vi "Plotter Keyvan.vi"() -> ()   [LabVIEW 2014]
panel:
  out "5":cluster{"Time":dbl[], "yi":dbl[]}[](graph)
  in  "Tab Control":enum32{"Graph 1", "Graph 2"}(tab)
  in  "RR":bool
  in  "RL":bool
  in  "FR":bool
  in  "FL":bool
  in  "RR":bool
  in  "RL":bool
  in  "FR":bool
  in  "FL":bool
  out "4":cluster{"Time":dbl[], "yi":dbl[]}[](graph)
  out "3":cluster{"Time":dbl[], "Vbb2":dbl[]}(graph)
  out "2":cluster{"Time":dbl[], "Vbb2":dbl[]}(graph)
  out "1":cluster{"Time":dbl[], "Vbb2":dbl[]}(graph)
  in  "Play Button":bool
  in  "Process Stop Button":bool
  in  "File path":path
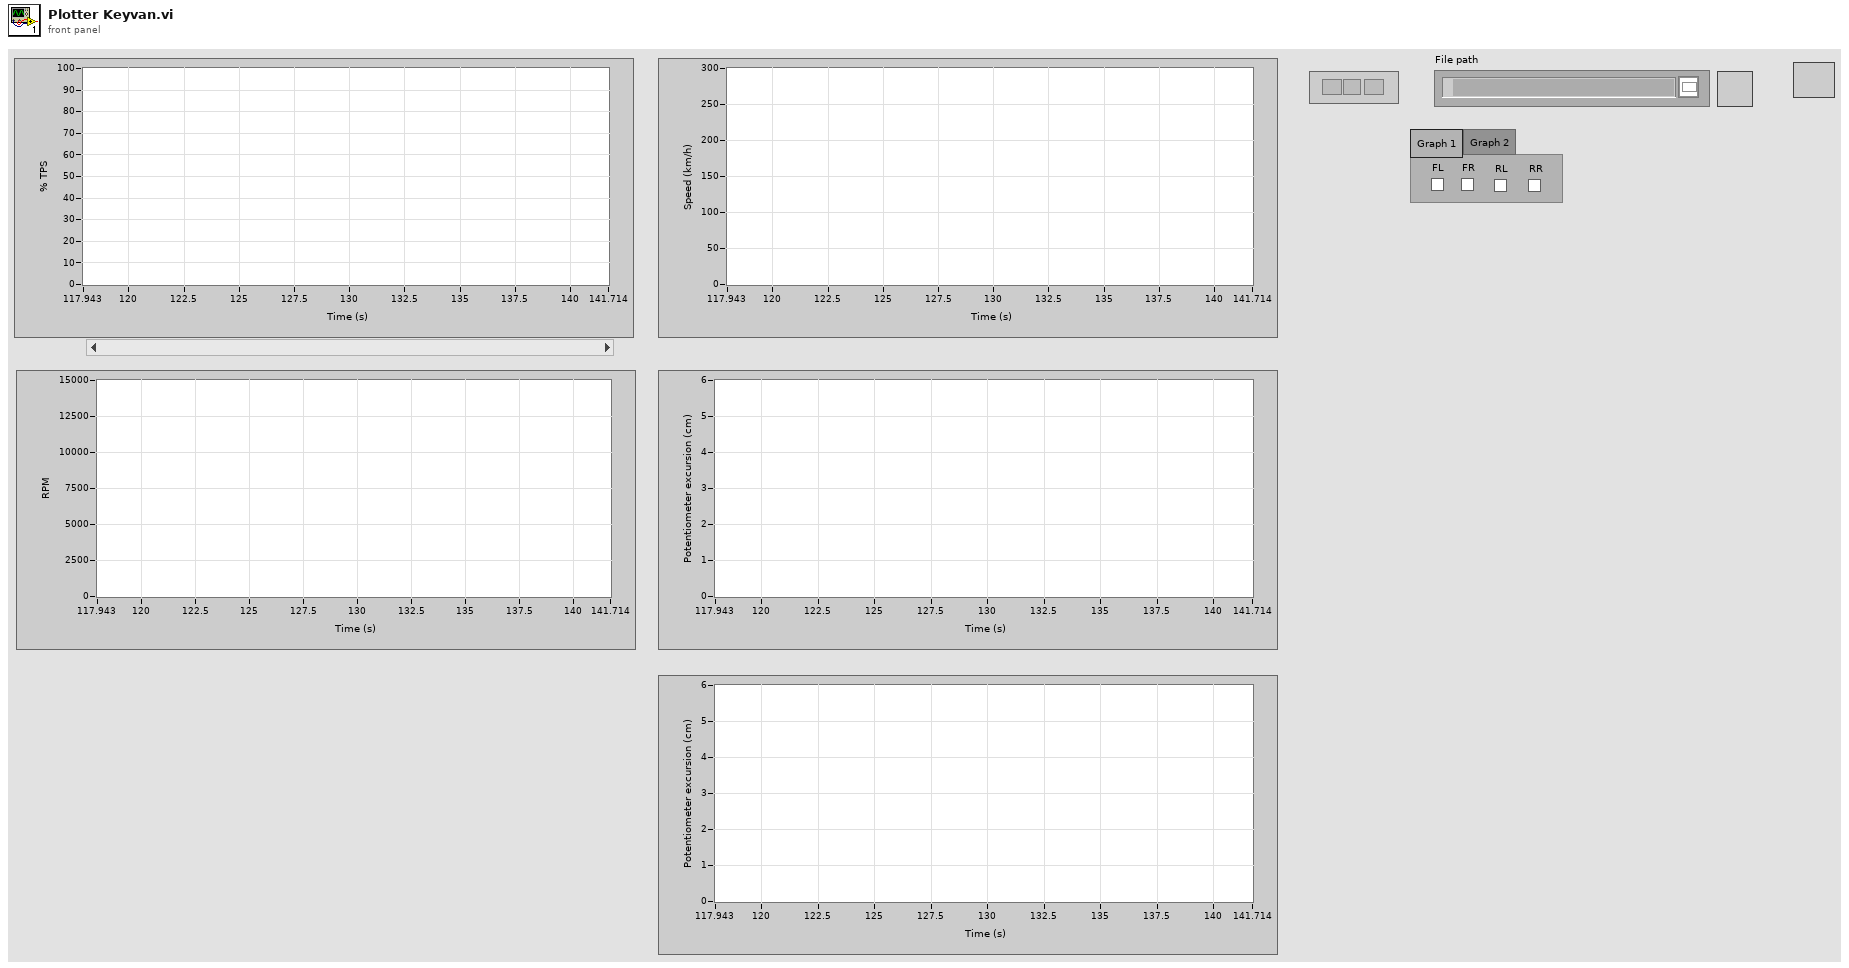
[diagram p1: front panel]
types:
  T1 = typedef "CAR Data Cluster.ctl" = cluster{"revs":dbl[], "rev/min":dbl[], "TPS":dbl[], "map":dbl[], "T H20":dbl[], "T Air":dbl[], "T Oil":dbl[], "Vbb1":dbl[], "Vbb2":dbl[], "Vbb3":dbl[], "Bar0":dbl[], "Lambda 1 AVG":dbl[], "Lambda 1 RAW":dbl[], "Lambda 2 AVG":dbl[], "Lambda 2 RAW":dbl[], "KLambda 1":dbl[], "KLambda 2":dbl[], "Inj Low":dbl[], "Spark 1":dbl[], "Phase Low":dbl[], "Phase High":dbl[], "Speed 1":dbl[], "Speed 2":dbl[], "DTPS+":dbl[], "DTPS-":dbl[], "DECAYINJ(+) - DECAYINJ(-)":dbl[], "DECAYIGN(+) - DECAYIGN(-)":dbl[], "Pot FL":dbl[], "Pot FR":dbl[], "Pot RL":dbl[], "Pot RR":dbl[], "Time":dbl[]}
  T2 = typedef "LVRangeTypeDef.ctl" = cluster{"Minimum":dbl, "Maximum":dbl, "Increment":dbl, "Minor Increment":dbl, "Start":dbl}
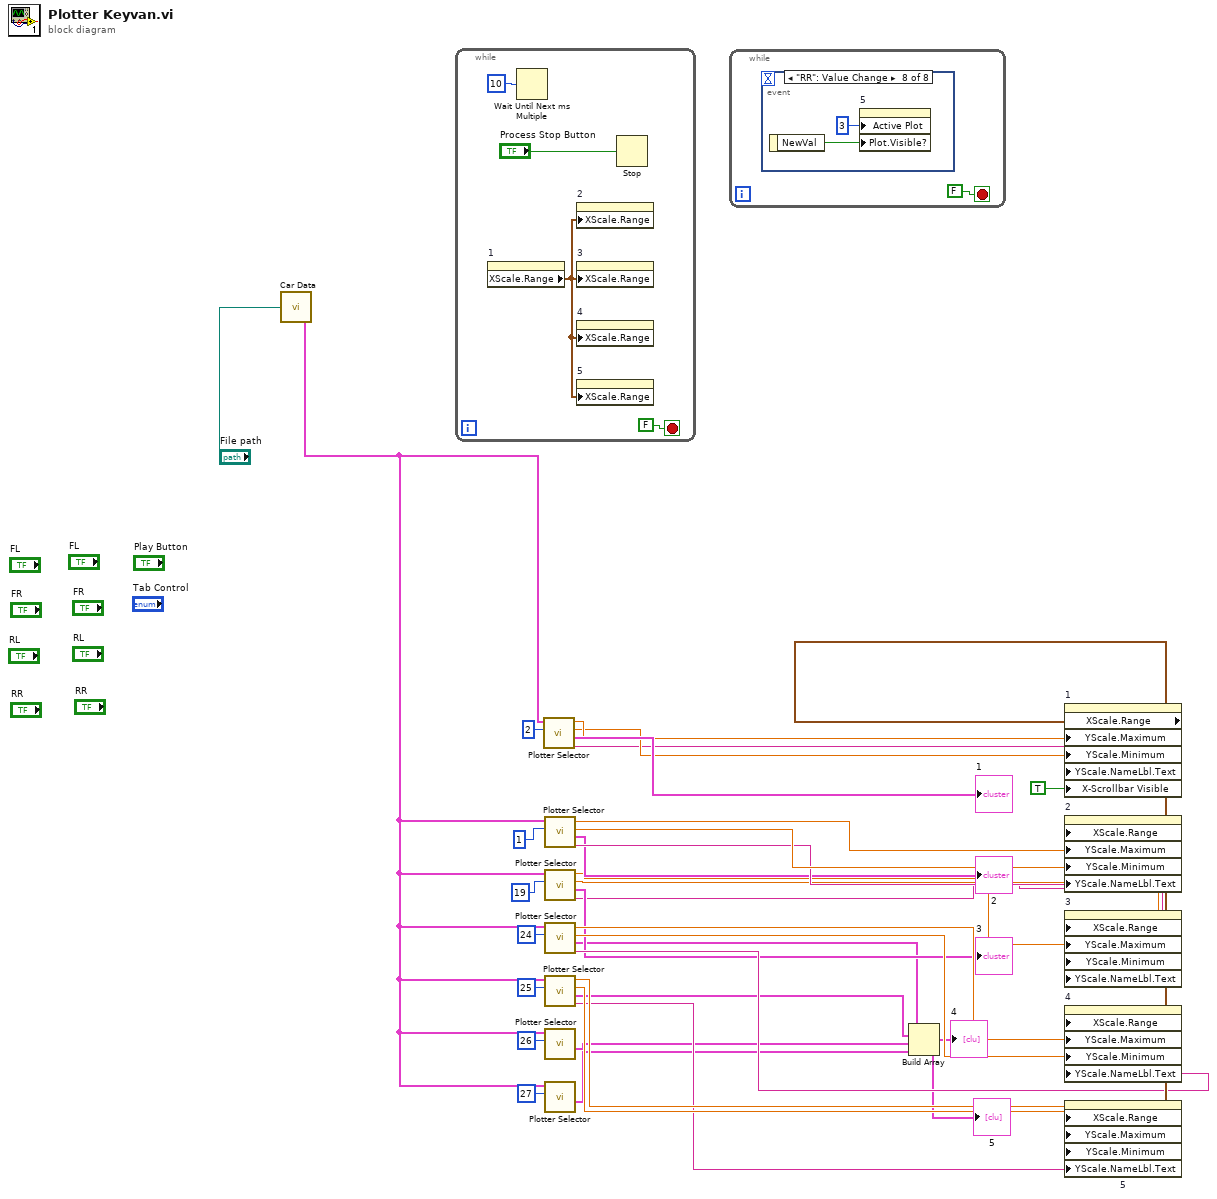
[diagram p0: block diagram]
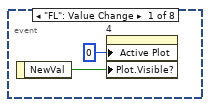
[diagram p2: hidden frame]
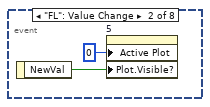
[diagram p3: hidden frame]
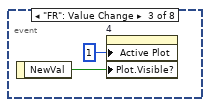
[diagram p4: hidden frame]
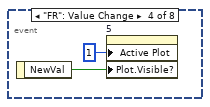
[diagram p5: hidden frame]
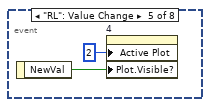
[diagram p6: hidden frame]
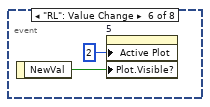
[diagram p7: hidden frame]
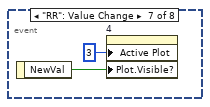
[diagram p8: hidden frame]
diagram:
  n1 = call "Car Data.vi"("file path (dialog if empty)"="File path") -> ("CAR DATA"=w27:T1)
  n2 = while {
    stop <- FALSE stop-if-true
    n3 = property on="1" class="XYGraph (strict)"() -> ("XScale.Range"=w35:T2)  [unwired: 2 in, 2 out]
    n4 = Wait Until Next ms Multiple(millisecond multiple=u32 10) -> ()  [unwired: 1 out]
    n5 = property on="2" class="XYGraph (strict)"("XScale.Range"=w35) -> ()  [unwired: 2 in, 2 out]
    n6 = property on="3" class="XYGraph (strict)"("XScale.Range"=w35) -> ()  [unwired: 2 in, 2 out]
    n7 = property on="4" class="XYGraph (strict)"("XScale.Range"=w35) -> ()  [unwired: 2 in, 2 out]
    n8 = property on="5" class="XYGraph (strict)"("XScale.Range"=w35) -> ()  [unwired: 2 in, 2 out]
    n9 = Stop(stop? (T)="Process Stop Button") -> ()
  }
  n10 = call "Plotter Selector.vi"("Ring Selector"=u16 2, "CAR DATA"=w27) -> ("Y Label"=w30:string, "Plot Output"=→"1":cluster{"Time":dbl[], "yi":dbl[]}, "Y Minimum"=w31:dbl, "Y Maximum"=w32:dbl)  [unwired: 6 in]
  n11 = call "Plotter Selector.vi"("Ring Selector"=u16 1, "CAR DATA"=w27) -> ("Y Label"=w18:string, "Plot Output"=→"2":cluster{"Time":dbl[], "yi":dbl[]}, "Y Minimum"=w20:dbl, "Y Maximum"=w19:dbl)  [unwired: 6 in]
  n12 = call "Plotter Selector.vi"("Ring Selector"=u16 19, "CAR DATA"=w27) -> ("Y Label"=w7:string, "Plot Output"=→"3":cluster{"Time":dbl[], "yi":dbl[]}, "Y Minimum"=w15:dbl, "Y Maximum"=w16:dbl)  [unwired: 6 in]
  n13 = call "Plotter Selector.vi"("Ring Selector"=u16 24, "CAR DATA"=w27) -> ("Y Label"=w9:string, "Plot Output"=w5:cluster{"Time":dbl[], "yi":dbl[]}, "Y Minimum"=w14:dbl, "Y Maximum"=w12:dbl)  [unwired: 6 in]
  n14 = call "Plotter Selector.vi"("Ring Selector"=u16 25, "CAR DATA"=w27) -> ("Y Label"=w6:string, "Plot Output"=w4:cluster{"Time":dbl[], "yi":dbl[]}, "Y Minimum"=w11:dbl, "Y Maximum"=w10:dbl)  [unwired: 6 in]
  n15 = call "Plotter Selector.vi"("Ring Selector"=u16 26, "CAR DATA"=w27) -> ("Plot Output"=w3:cluster{"Time":dbl[], "yi":dbl[]})  [unwired: 6 in, 3 out]
  n16 = call "Plotter Selector.vi"("Ring Selector"=u16 27, "CAR DATA"=w27) -> ("Plot Output"=w2:cluster{"Time":dbl[], "yi":dbl[]})  [unwired: 6 in, 3 out]
  n17 = while {
    stop <- FALSE stop-if-true
    n18 = event shown="[7] \"RR\": Value Change" {
      selector: _ -> [_ _ _ _ _ _ _ _]
      dyn-events: _ -> [_ _ _ _ _ _ _ _]
      timeout: _ -> [_ _ _ _ _ _ _ _]
      event "FL": Value Change {
        n19 = event-data() -> ("NewVal"=w40:bool)  [unwired: 1 in]
        n20 = property on="4" class="XYGraph (strict)"("Active Plot"=u32 0, "Plot.Visible?"=w40) -> ()  [unwired: 2 in, 2 out]
      }
      event "FL": Value Change {
        n21 = event-data() -> ("NewVal"=w42:bool)  [unwired: 1 in]
        n22 = property on="5" class="XYGraph (strict)"("Active Plot"=u32 0, "Plot.Visible?"=w42) -> ()  [unwired: 2 in, 2 out]
      }
      event "FR": Value Change {
        n23 = event-data() -> ("NewVal"=w44:bool)  [unwired: 1 in]
        n24 = property on="4" class="XYGraph (strict)"("Active Plot"=u32 1, "Plot.Visible?"=w44) -> ()  [unwired: 2 in, 2 out]
      }
      event "FR": Value Change {
        n25 = event-data() -> ("NewVal"=w46:bool)  [unwired: 1 in]
        n26 = property on="5" class="XYGraph (strict)"("Active Plot"=u32 1, "Plot.Visible?"=w46) -> ()  [unwired: 2 in, 2 out]
      }
      event "RL": Value Change {
        n27 = event-data() -> ("NewVal"=w48:bool)  [unwired: 1 in]
        n28 = property on="4" class="XYGraph (strict)"("Active Plot"=u32 2, "Plot.Visible?"=w48) -> ()  [unwired: 2 in, 2 out]
      }
      event "RL": Value Change {
        n29 = event-data() -> ("NewVal"=w50:bool)  [unwired: 1 in]
        n30 = property on="5" class="XYGraph (strict)"("Active Plot"=u32 2, "Plot.Visible?"=w50) -> ()  [unwired: 2 in, 2 out]
      }
      event "RR": Value Change {
        n31 = event-data() -> ("NewVal"=w53:bool)  [unwired: 1 in]
        n32 = property on="4" class="XYGraph (strict)"("Active Plot"=u32 3, "Plot.Visible?"=w53) -> ()  [unwired: 2 in, 2 out]
      }
      event "RR": Value Change {
        n33 = event-data() -> ("NewVal"=w55:bool)  [unwired: 1 in]
        n34 = property on="5" class="XYGraph (strict)"("Active Plot"=u32 3, "Plot.Visible?"=w55) -> ()  [unwired: 2 in, 2 out]
      }
    }
  }
  n35 = Build Array(w5, w4, w3, w2) -> (→"4" →"5":cluster{"Time":dbl[], "yi":dbl[]}[])
  n36 = property on="1" class="XYGraph (strict)"("YScale.Maximum"=w32, "YScale.Minimum"=w31, "YScale.NameLbl.Text"=w30, "X-Scrollbar Visible"=TRUE ("X Scrollbar Visible")) -> ("XScale.Range"=w13:T2)  [unwired: 2 in, 2 out]
  n37 = property on="2" class="XYGraph (strict)"("XScale.Range"=w13, "YScale.Maximum"=w19, "YScale.Minimum"=w20, "YScale.NameLbl.Text"=w18) -> ()  [unwired: 2 in, 2 out]
  n38 = property on="3" class="XYGraph (strict)"("XScale.Range"=w13, "YScale.Maximum"=w16, "YScale.Minimum"=w15, "YScale.NameLbl.Text"=w7) -> ()  [unwired: 2 in, 2 out]
  n39 = property on="4" class="XYGraph (strict)"("XScale.Range"=w13, "YScale.Maximum"=w12, "YScale.Minimum"=w14, "YScale.NameLbl.Text"=w9) -> ()  [unwired: 2 in, 2 out]
  n40 = property on="5" class="XYGraph (strict)"("XScale.Range"=w13, "YScale.Maximum"=w10, "YScale.Minimum"=w11, "YScale.NameLbl.Text"=w6) -> ()  [unwired: 2 in, 2 out]
